vi "test Should Return Parameters from First and Last Call.vi"(8 "error in (no error)":errorcluster, 11 "TestCase in":refnum<class "Store and Return Parameters.lvclass">) -> (0 "error out":errorcluster, 3 "TestCase out":refnum<class "Store and Return Parameters.lvclass">)   [LabVIEW 2013, in "Store and Return Parameters.lvclass"]
uses:
  Store and Return Parameters.lvclass
  Core Classes/LabSpy/LabSpy.lvclass
  <vilib>/addons/_JKI Toolkits/VI Tester/TestCase.llb/TestCase.lvclass
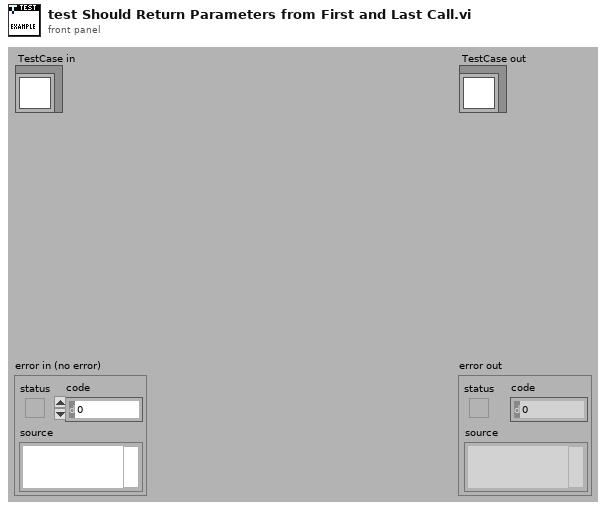
[diagram p1: front panel]
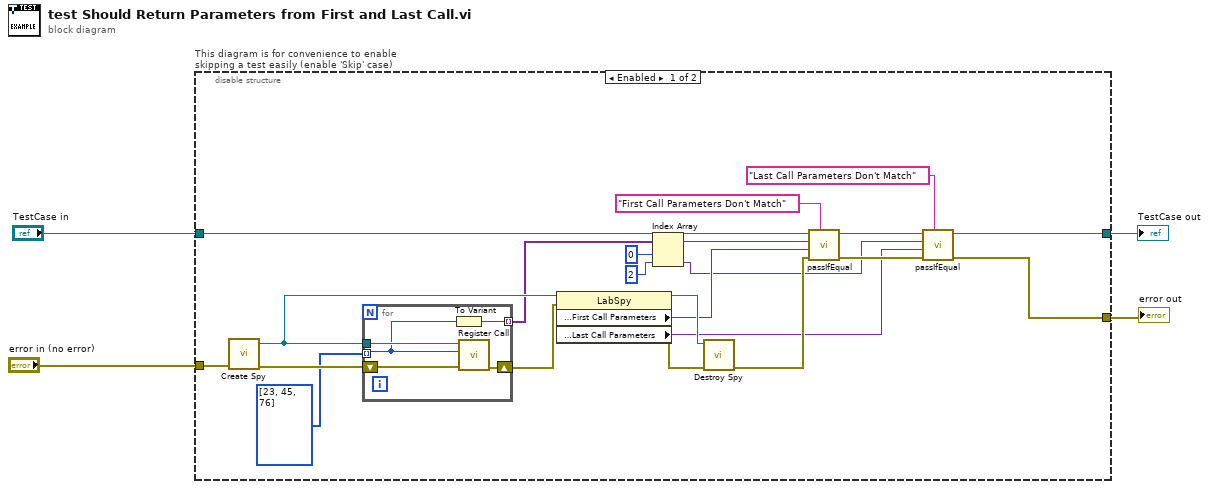
[diagram p0: block diagram]
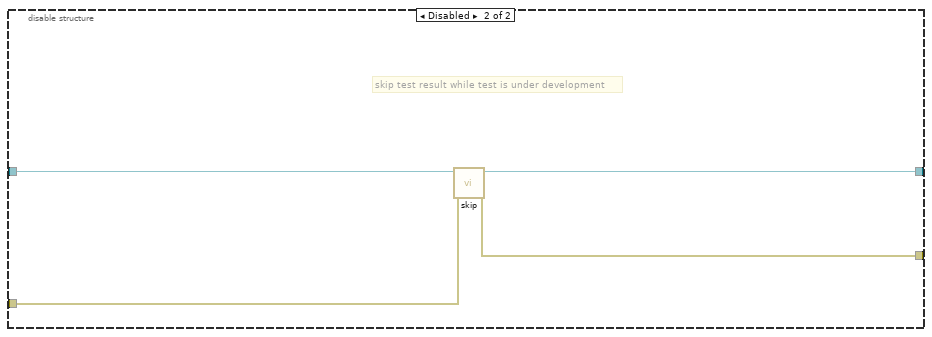
[diagram p2: hidden frame]
diagram:
  n1 = disable-structure "This diagram is for convenience to enable skipping a test easily (enable 'Skip' case)" shown="Enabled" {
    disable-tunnel: "TestCase in" -> [w20 w35]
    disable-tunnel: [w10 w33] -> w1
    disable-tunnel: [w12 w34] -> w3
    disable-tunnel: "error in (no error)" -> [w26 w32]
    frame Enabled {
      n2 = call "Create Spy.vi"("error in (no error)"=w26) -> ("error out"=w25:errorcluster, "LabSpy Out"=w24:refnum<data-value>)  [unwired: 9 in]
      n3 = for {
        tunnel: w24 -> [w30]
        shift-right: [w29] -> w23
        shift-left: w25 -> [w31]
        tunnel: i32[] [23, 45, 76] -> [w28] mode=indexing
        tunnel: [w27] -> w15 mode=indexing
        n4 = To Variant(anything=w28) -> (Variant=w27:variant)
        n5 = call "Register Call.vi"("error in (no error)"=w31, "Parameters"=w28, "LabSpy"=w30) -> ("error out"=w29:errorcluster)  [unwired: 7 in, 1 out]
      }
      n6 = property class="LabSpy"(reference=w24, error in=w23) -> (reference out=w21:refnum<data-value>, error out=w22:errorcluster, "Parameter Readings:First Call Parameters"=w17:variant, "Parameter Readings:Last Call Parameters"=w9:variant)
      n7 = Index Array(array=w15, index #1=0 ("index"), index #2=2 ("index")) -> (element #1=w14:variant, element #2=w8:variant)
      n8 = call "Destroy Spy.vi"("error in (no error)"=w22, "LabSpy"=w21) -> ("error out"=w18:errorcluster)  [unwired: 9 in]
      n9 = call-dynamic "passIfEqual.vi"("custom report message (\"\")"="First Call Parameters Don't Match" ("custom report message (\"\")"), "error in (no error)"=w18, "y"=w17, "x"=w14, "TestCase in"=w20) -> ("error out"=w19:errorcluster, "TestCase out"=w11:refnum<class "Store and Return Parameters.lvclass">)  [unwired: 5 in]
      n10 = call-dynamic "passIfEqual.vi"("custom report message (\"\")"="Last Call Parameters Don't Match" ("custom report message (\"\")"), "error in (no error)"=w19, "y"=w9, "x"=w8, "TestCase in"=w11) -> ("error out"=w12:errorcluster, "TestCase out"=w10:refnum<class "Store and Return Parameters.lvclass">)  [unwired: 5 in]
    }
    frame Disabled {
      # "skip test result while test is under development"
      n11 = call <vilib>:"skip.vi"("error in (no error)"=w32, "TestCase in"=w35) -> ("error out"=w34:errorcluster, "TestCase out"=w33:refnum<class "Store and Return Parameters.lvclass">)  [unwired: 8 in]
    }
  }
  "error out" <- w3
  "TestCase out" <- w1
